vi "PDE_State_Machine_12_12_ver_3.vi"() -> ()   [LabVIEW 2017]
uses:
  SubVIs/FireSlider.ctl
  StateIndicator.ctl
  PDEState.ctl
  <vilib>/DAQmx/write.llb/DAQmx Write (Digital 1D Wfm NChan NSamp).vi
  <vilib>/DAQmx/read.llb/DAQmx Read (Analog 1D Wfm NChan NSamp).vi
  <vilib>/DAQmx/write.llb/DAQmx Write (Digital Wfm 1Chan NSamp).vi
  <vilib>/DAQmx/write.llb/DAQmx Write (Digital Bool 1Line 1Point).vi
  <vilib>/DAQmx/create/channels.llb/DAQmx Create Channel (AI-Current-Basic).vi
  <vilib>/DAQmx/create/channels.llb/DAQmx Create Channel (AI-Voltage-Basic).vi
  <vilib>/DAQmx/configure/timing.llb/DAQmx Timing (Sample Clock).vi
  <vilib>/DAQmx/create/channels.llb/DAQmx Create Channel (DO-Digital Output).vi
  <vilib>/DAQmx/create/channels.llb/DAQmx Create Channel (AI-Temperature-Thermocouple).vi
  <vilib>/Waveform/DWDTOps.llb/DWDT Uncompress Digital.vi
  <vilib>/DAQmx/miscellaneous.llb/DAQmx Fill In Error Info.vi
  <vilib>/Waveform/DTblOps.llb/DTbl Boolean Array to Digital.vi
  <resource>/objmgr/daqmx.rc
panel:
  out "PDE Sensors 2":T1 {"Downstream Oxygen" scale=0.0..150.0; "Upstream Oxygen" scale=0.0..150.0; "Fuel Pressure" scale=0.0..150.0}
  out "Predet Sensors 2":T2 {"Fuel Pressure" scale=0.0..150.0; "Oxidizer Pressure" scale=0.0..150.0}
  in  "Set_Oxygen_Pressure":bool
  in  "Save Data":bool
  in  "Filename":path=path "test.tdms"
  out "PDE Sensors":T1 {"Downstream Oxygen" scale=0.0..150.0; "Upstream Oxygen" scale=0.0..150.0; "Fuel Pressure" scale=0.0..150.0}
  in  "Predet Freq (Hz)":dbl=20.0 format="%#_13g"
  out "Predet Sensors":T2 {"Fuel Pressure" scale=0.0..150.0; "Oxidizer Pressure" scale=0.0..150.0}
  out "PDE Progress":dbl(slide) scale=0.0..1.0
  out "Predet Progress":dbl(slide) scale=0.0..1.0
  in  "Number of Predet Fires":T3=1 min=0 max=100 step=1 scale=1.0..100.0
  out "Predet Fire Counter":i32
  out "PDE State":T4 items=["Stop VI", "Predet Fire", "Control Button", "Stop", "Connecting", "Firing", "Testing ", "Idle", "Init"]
  in  "Number of Fires":T3=1 min=0 max=100 step=1 scale=1.0..100.0
  out "Fire Counter":i32
  in  "Predet Fire Button":bool
  in  "PDE Fire Button":bool
  in  "Test Button":bool
  in  "Go To Idle":bool
  in  "Abort VI":bool
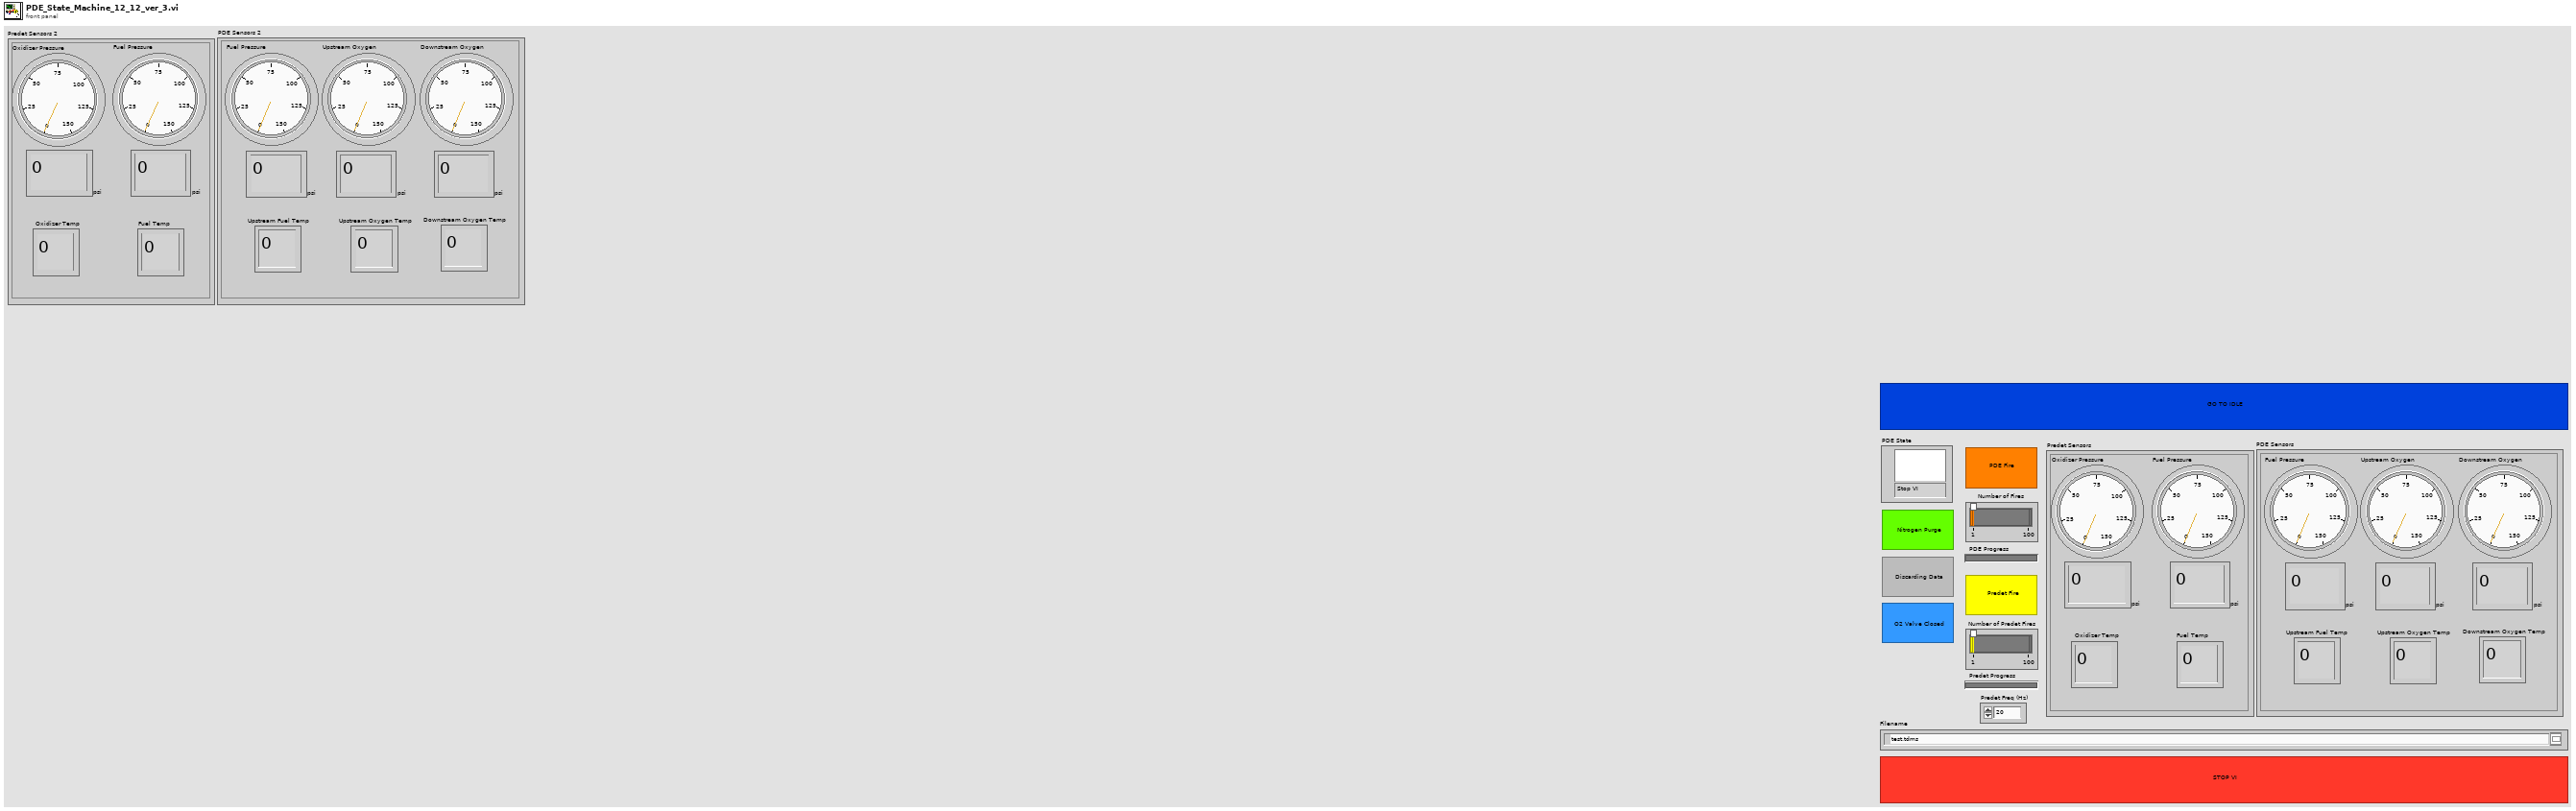
[diagram p1: front panel]
types:
  T1 = cluster{"Fuel Pressure":dbl, "Upstream Oxygen ":dbl, "Downstream Oxygen ":dbl, "Oxidizer Temp":dbl, "Oxidizer Temp 2":dbl, "Oxidizer Temp 3":dbl}
  T2 = cluster{"Oxidizer Pressure":dbl, "Fuel Pressure":dbl, "Oxidizer Temp":dbl, "Fuel Temp":dbl}
  T3 = typedef "FireSlider.ctl" = i32
  T4 = typedef "StateIndicator.ctl" = u16
  T5 = typedef "PDEState.ctl" = enum16{"Stop VI", "Predet Fire", "Control Button", "Stop", "Connecting", "Firing ", "Testing ", "Idle", "Init"}
  T6 = cluster{"Scalar":dbl, "Scalar":dbl, "Scalar":dbl, "Scalar":dbl, "Scalar":dbl, "Scalar":dbl}
  T7 = cluster{"Scalar":dbl, "Scalar":dbl, "Scalar":dbl, "Scalar":dbl}
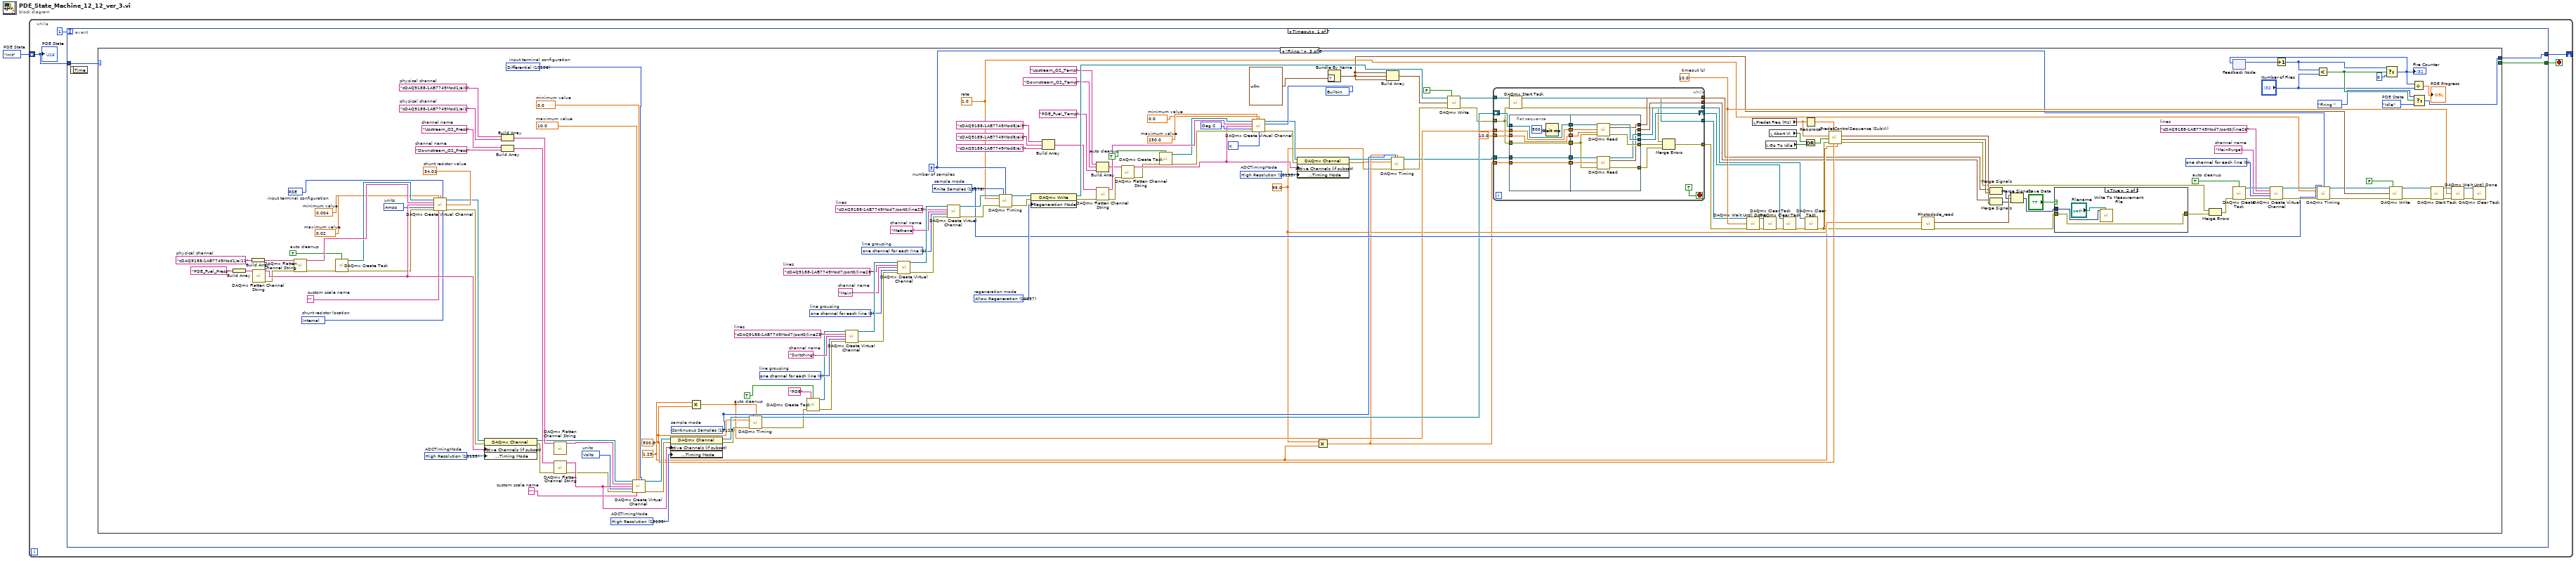
[diagram p0: block diagram]
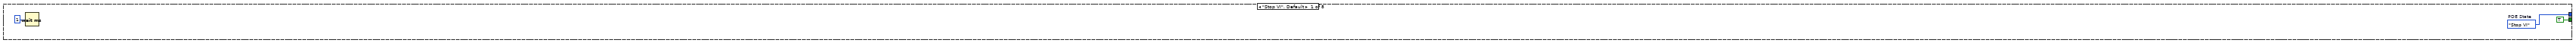
[diagram p2: hidden frame]
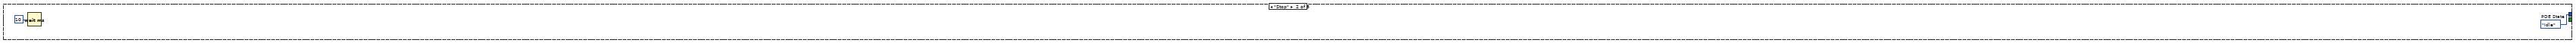
[diagram p3: hidden frame]
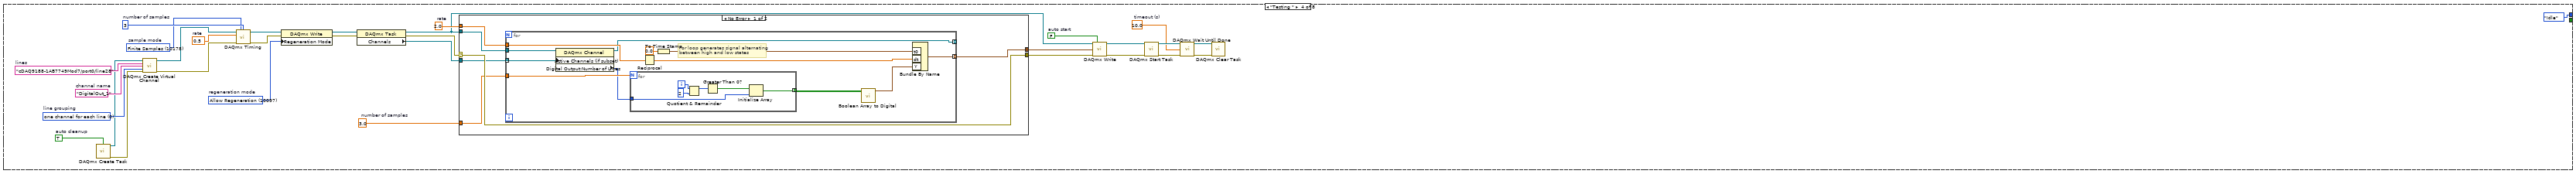
[diagram p5: hidden frame]
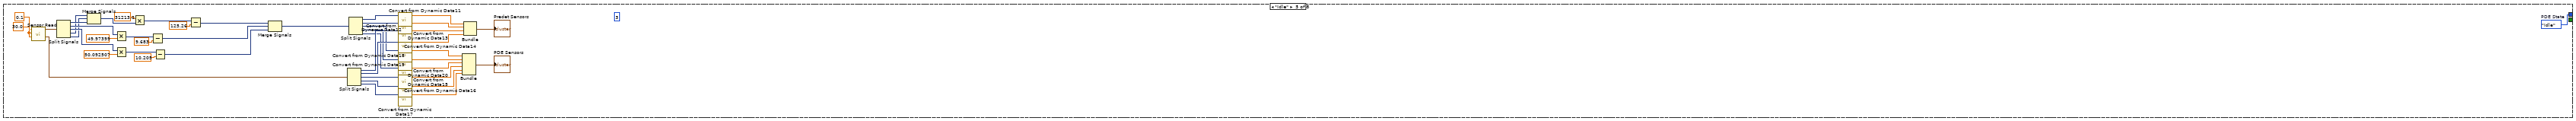
[diagram p7: hidden frame]
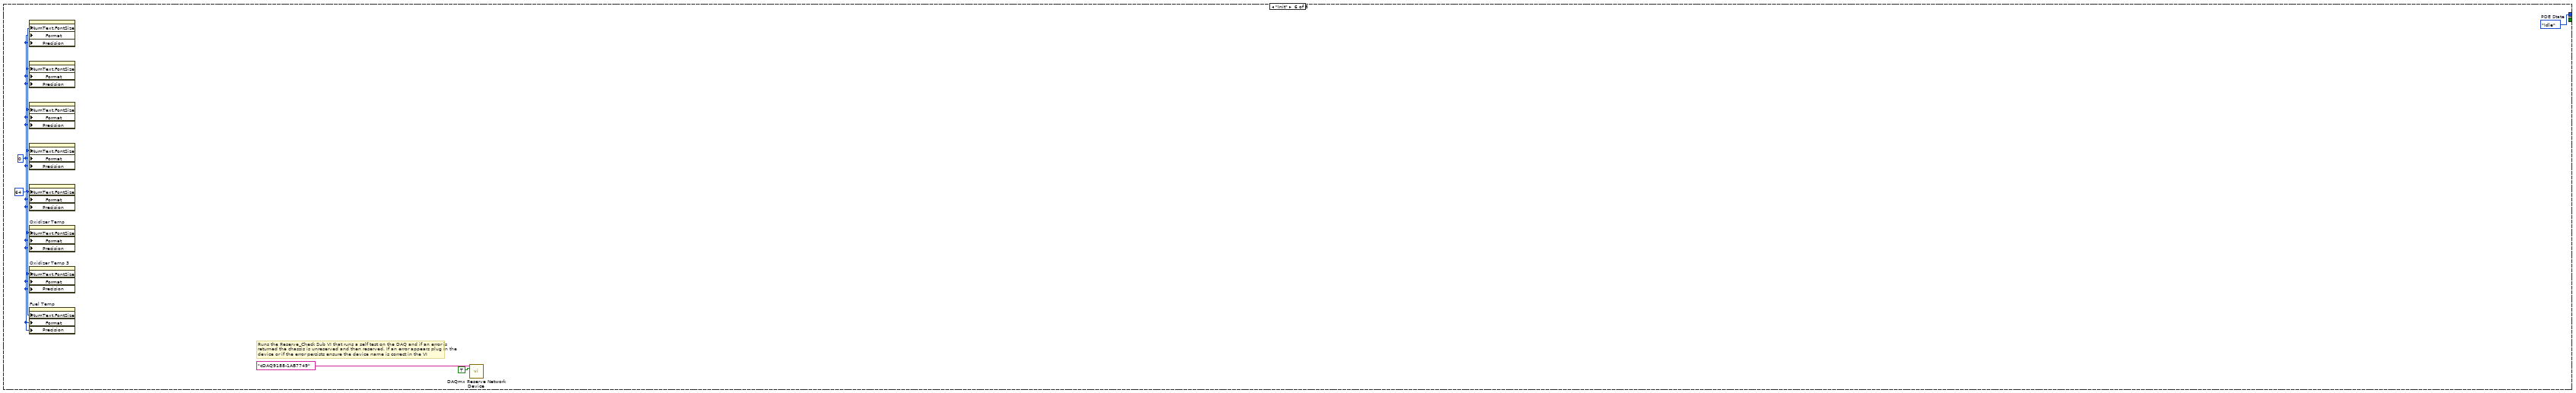
[diagram p8: hidden frame]
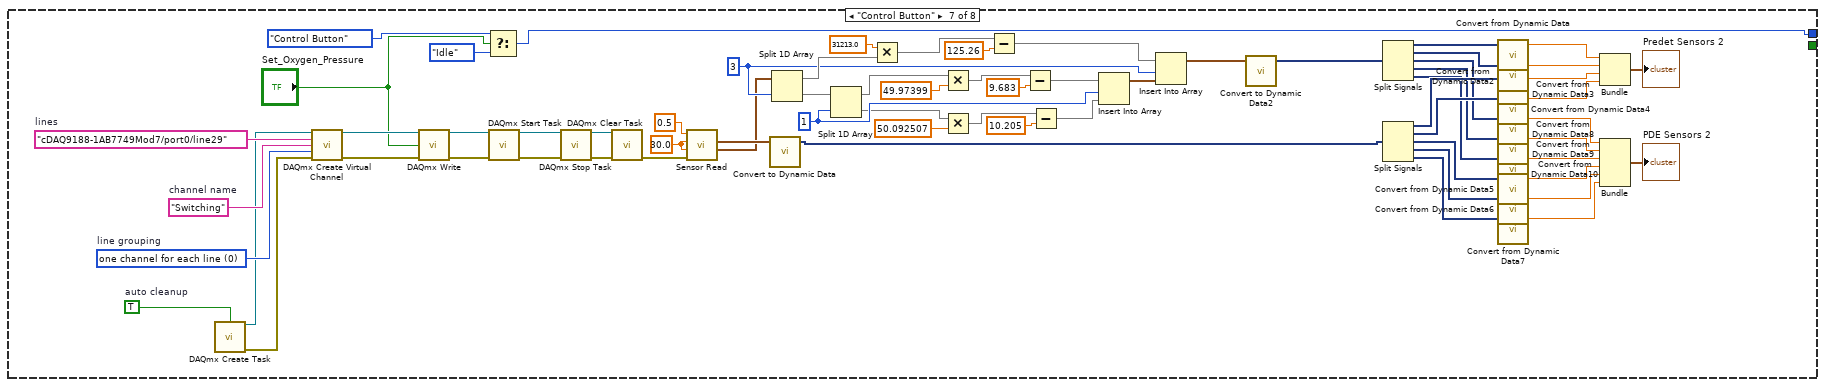
[diagram p9: hidden frame]
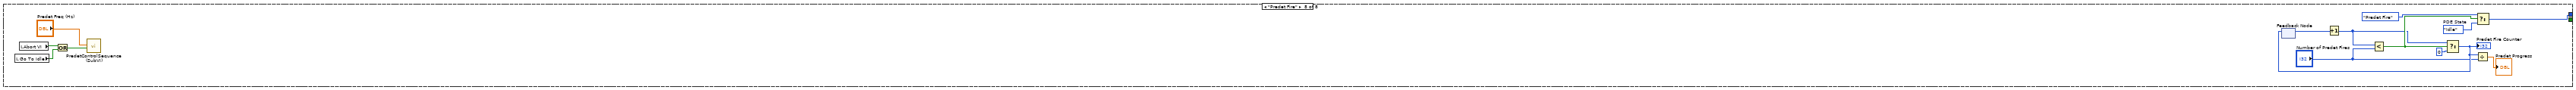
[diagram p10: hidden frame]
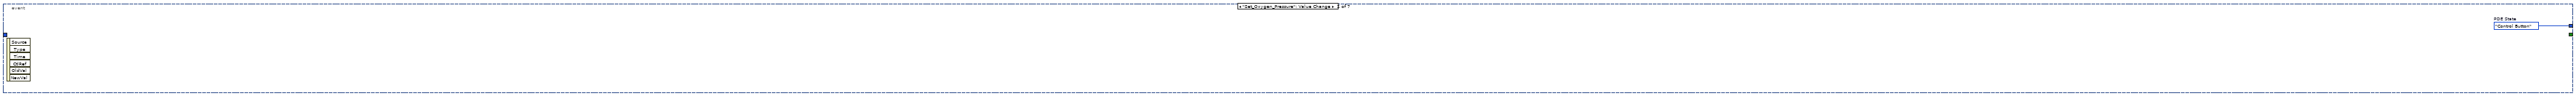
[diagram p11: hidden frame]
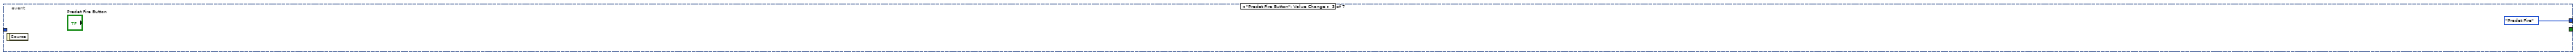
[diagram p12: hidden frame]
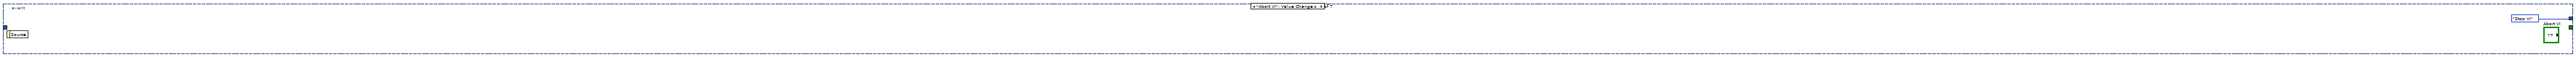
[diagram p13: hidden frame]
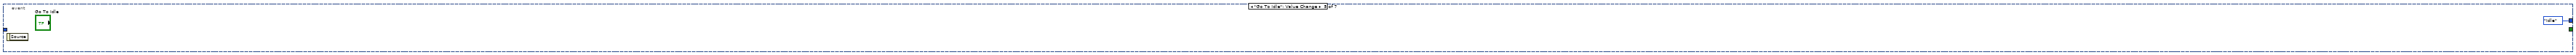
[diagram p14: hidden frame]
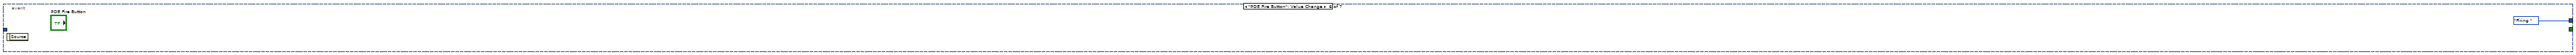
[diagram p15: hidden frame]
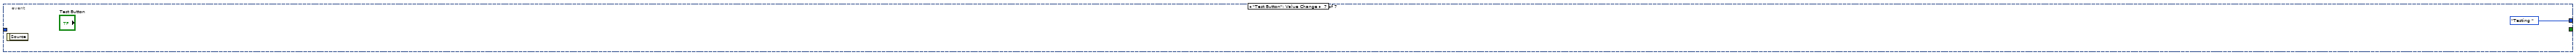
[diagram p16: hidden frame]
diagram:
  w1 = PDEState."Init"  # PDE State
  n1 = while {
    shift-right: [w4] -> _
    shift-left: w1 -> [w2]
    stop <- w3 stop-if-true
    n2 = event shown="[0] Timeout" {
      selector: _ -> [_ _ _ _ _ _ _]
      dyn-events: _ -> [_ _ _ _ _ _ _]
      timeout: 1 -> [_ _ _ _ _ _ _]
      tunnel: w2 -> [w8 _ _ _ _ _ _]
      tunnel: [w7 w415 PDEState."Predet Fire" ("PDE State") PDEState."Stop VI" ("PDE State") PDEState."Idle" ("PDE State") PDEState."Firing " ("PDE State") PDEState."Testing " ("PDE State")] -> w4
      tunnel: [w6 _ _ _ _ _ _] -> w3
      event Timeout {
        n3 = event-data() -> ()  [unwired: 1 in, 1 out]
        n4 = case shown="\"Firing \"" w8 {
          tunnel: [w11 w13 w175 PDEState."Idle" ("PDE State") w328 w333 w399 w408] -> w7
          tunnel: [TRUE _ _ _ _ _ _ _] -> w6
          frame "Stop VI", Default {
            w11 = PDEState."Stop VI"  # PDE State
            n5 = Wait (ms)(milliseconds to wait=u32 1 ("millisecond timer value")) -> ()  [unwired: 1 out]
          }
          frame "Stop" {
            w13 = PDEState."Idle"  # PDE State
            n6 = Wait (ms)(milliseconds to wait=u32 10 ("millisecond timer value")) -> ()  [unwired: 1 out]
          }
          frame "Firing " {
            w89 = 10195 items=["High Resolution"=10195, "High Speed"=14712, "Best 50 Hz Rejection"=14713, "Best 60 Hz Rejection"=14714]  # ADCTimingMode
            w100 = "Downstream_O2_Press"  # channel name
            w97 = "cDAQ9188-1AB7749Mod1/ai1"  # physical channel
            w88 = 10106 items=["default"=-1, "RSE"=10083, "NRSE"=10078, "Differential"=10106, "Pseudodifferential"=12529]  # input terminal configuration
            w102 = 10348 items=["Volts"=10348, "From Custom Scale"=10065]  # units
            w101 = "Upstream_O2_Press"  # channel name
            w87 = ""  # custom scale name
            w86 = 0.0  # minimum value
            w85 = 10.0  # maximum value
            w96 = "cDAQ9188-1AB7749Mod1/ai0"  # physical channel
            w83 = "cDAQ9188-1AB7749Mod1/ai11"  # physical channel
            w90 = 10123 items=["Finite Samples"=10178, "Continuous Samples"=10123, "Hardware Timed Single Point"=12522]  # sample mode
            w63 = 10195 items=["High Resolution"=10195, "High Speed"=14712, "Best 50 Hz Rejection"=14713, "Best 60 Hz Rejection"=14714]  # ADCTimingMode
            w64 = 10083 items=["default"=-1, "RSE"=10083, "NRSE"=10078, "Differential"=10106, "Pseudodifferential"=12529]  # input terminal configuration
            w65 = 10342 items=["Amps"=10342, "From Custom Scale"=10065]  # units
            w66 = 34.01  # shunt resistor value
            w67 = 10200 items=["Internal"=10200, "External"=10167]  # shunt resistor location
            w69 = ""  # custom scale name
            w70 = 0.004  # minimum value
            w71 = 0.02  # maximum value
            w73 = TRUE  # auto cleanup
            w60 = 10143 items=["Deg C"=10143, "Deg F"=10144, "Kelvins"=10325, "Deg R"=10145, "From Custom Scale"=10065] ("units")
            w59 = 10073 items=["J"=10072, "K"=10073, "N"=10077, "R"=10082, "S"=10085, "T"=10086, "B"=10047, "E"=10055] ("thermocouple type")
            w58 = 10200 items=["Built-In"=10200, "Constant Value"=10116, "Channel"=10113] ("cjc source")
            w49 = 10195 items=["High Resolution"=10195, "High Speed"=14712, "Best 50 Hz Rejection"=14713, "Best 60 Hz Rejection"=14714]  # ADCTimingMode
            w52 = 0.0  # minimum value
            w53 = 250.0  # maximum value
            w55 = TRUE  # auto cleanup
            w34 = 1.25 ("Sampling Time")
            w35 = 95.0 ("Temperature Freq")
            w36 = 500.0 ("Pressure Freq")
            w130 = 0 items=["one channel for each line", "one channel for all lines"] ("line grouping")
            w136 = 0 items=["one channel for each line", "one channel for all lines"]  # line grouping
            w135 = "Methane"  # channel name
            w137 = "cDAQ9188-1AB7749Mod7/port0/line25"  # lines
            w141 = 0 items=["one channel for each line", "one channel for all lines"]  # line grouping
            w140 = "Main"  # channel name
            w142 = "cDAQ9188-1AB7749Mod7/port0/line28"  # lines
            w146 = 0 items=["one channel for each line", "one channel for all lines"]  # line grouping
            w145 = "Switching"  # channel name
            w147 = "cDAQ9188-1AB7749Mod7/port0/line29"  # lines
            w161 = TRUE  # auto cleanup
            w156 = "MainPurge"  # channel name
            w157 = "cDAQ9188-1AB7749Mod7/port0/line26"  # lines
            w168 = 10097 items=["Allow Regeneration"=10097, "Do Not Allow Regeneration"=10158]  # regeneration mode
            w123 = 10178 items=["Finite Samples"=10178, "Continuous Samples"=10123, "Hardware Timed Single Point"=12522]  # sample mode
            w124 = 3  # number of samples
            w122 = 1.0  # rate
            w170 = TRUE  # auto cleanup
            w148 = 10.0  # timeout (s)
            w176 = PDEState."Idle"  # PDE State
            n7 = Build Array("PDE_Fuel_Press" ("element")) -> (w76:string[])
            n8 = Build Array(w83) -> (w78:string[])
            n9 = call <vilib>:"DAQmx Flatten Channel String.vi"("names in"=w76) -> ("names out"=w77:string, "error out"=w38:errorcluster)  [unwired: 13 in]
            n10 = call <vilib>:"DAQmx Flatten Channel String.vi"("names in"=w78, "error in"=w38) -> ("names out"=w75:string, "error out"=w16:errorcluster)  [unwired: 12 in]
            n11 = call <vilib>:"DAQmx Create Task.vi"("auto cleanup"=w73, "error in"=w16) -> ("task out"=w72:refnum<k21>, "error out"=w74:errorcluster)  [unwired: 3 in, 9 out]
            n12 = call-poly <vilib>:"DAQmx Create Virtual Channel.vi"("task in"=w72, "maximum value"=w71, "minimum value"=w70, "input terminal configuration"=w64, "physical channels"=w75, "name to assign"=w77, "external shunt resistor value"=w66, "units"=w65, "error in"=w74, "custom scale name"=w69, "shunt resistor location"=w67) -> ("task out"=w62:refnum<k21>, "error out"=w68:errorcluster)  [unwired: 3 out]
            n13 = property class="DAQmx Channel"(reference=w62, error in=w68, "Active Channels (if subset)"=w77, "Analog Input:General Properties:Digitizer/ADC:Timing Mode"=w63) -> (reference out=w92:refnum<k21>, error out=w18:errorcluster)
            n14 = Build Array(w96, w97) -> (w95:string[])
            n15 = Build Array(w101, w100) -> (w99:string[])
            n16 = call <vilib>:"DAQmx Flatten Channel String.vi"("names in"=w95) -> ("names out"=w98:string)  [unwired: 13 in, 1 out]
            n17 = call <vilib>:"DAQmx Flatten Channel String.vi"("names in"=w99, "error in"=w18) -> ("names out"=w105:string, "error out"=w17:errorcluster)  [unwired: 12 in]
            n18 = call-poly <vilib>:"DAQmx Create Virtual Channel.vi"("task in"=w92, "maximum value"=w85, "minimum value"=w86, "input terminal configuration"=w88, "physical channels"=w98, "name to assign"=w105, "units"=w102, "error in"=w17, "custom scale name"=w87) -> ("task out"=w103:refnum<k21>, "error out"=w104:errorcluster)  [unwired: 5 in]
            n19 = property class="DAQmx Channel"(reference=w103, error in=w104, "Active Channels (if subset)"=w105, "Analog Input:General Properties:Digitizer/ADC:Timing Mode"=w89) -> (reference out=w91:refnum<k21>, error out=w93:errorcluster)
            n20 = Multiply(x=w34, y=w36) -> (x*y=w39:dbl)
            n21 = call-poly <vilib>:"DAQmx Timing.vi"("task/channels in"=w91, "sample mode"=w90, "samples per channel"=w39, "rate"=w36, "error in"=w93) -> ("task out"=w79:refnum<k21>, "error out"=w22:errorcluster)  [unwired: 2 in, 7 out]
            n22 = call <vilib>:"DAQmx Create Task.vi"("new task name"="PDE", "auto cleanup"=w170, "error in"=w22) -> ("task out"=w131:refnum<k21>, "error out"=w132:errorcluster)  [unwired: 11 in]
            n23 = call-poly <vilib>:"DAQmx Create Virtual Channel.vi"("task in"=w131, "lines"=w147, "name to assign"=w145, "line grouping"=w146, "error in"=w132) -> ("task out"=w143:refnum<k21>, "error out"=w144:errorcluster)  [unwired: 9 in]
            n24 = call-poly <vilib>:"DAQmx Create Virtual Channel.vi"("task in"=w143, "lines"=w142, "name to assign"=w140, "line grouping"=w141, "error in"=w144) -> ("task out"=w138:refnum<k21>, "error out"=w139:errorcluster)  [unwired: 9 in]
            n25 = call-poly <vilib>:"DAQmx Create Virtual Channel.vi"("task in"=w138, "lines"=w137, "name to assign"=w135, "line grouping"=w136, "error in"=w139) -> ("task out"=w133:refnum<k21>, "error out"=w134:errorcluster)  [unwired: 9 in]
            n26 = call-poly <vilib>:"DAQmx Timing.vi"("task/channels in"=w133, "sample mode"=w123, "samples per channel"=w124, "rate"=w122, "error in"=w134) -> ("task out"=w169:refnum<k21>, "error out"=w21:errorcluster)  [unwired: 9 in]
            n27 = property class="DAQmx Write"(reference=w169, error in=w21, "Regeneration Mode"=w168) -> (reference out=w167:refnum<k21>, error out=w20:errorcluster)
            n28 = Build Array("cDAQ9188-1AB7749Mod8/ai5" ("element"), "cDAQ9188-1AB7749Mod8/ai6" ("element"), "cDAQ9188-1AB7749Mod8/ai7" ("element")) -> (w61:string[])
            n29 = Build Array("Upstream_O2_Temp" ("name to assign"), "Downstream_O2_Temp" ("name to assign"), "PDE_Fuel_Temp" ("name to assign")) -> (w45:string[])
            n30 = call <vilib>:"DAQmx Flatten Channel String.vi"("names in"=w61, "error in"=w20) -> ("names out"=w57:string, "error out"=w37:errorcluster)  [unwired: 12 in]
            n31 = call <vilib>:"DAQmx Flatten Channel String.vi"("names in"=w45, "error in"=w37) -> ("names out"=w41:string, "error out"=w40:errorcluster)  [unwired: 12 in]
            n32 = call <vilib>:"DAQmx Create Task.vi"("auto cleanup"=w55, "error in"=w40) -> ("task out"=w54:refnum<k21>, "error out"=w56:errorcluster)  [unwired: 3 in, 9 out]
            n33 = call-poly <vilib>:"DAQmx Create Virtual Channel.vi"("task in"=w54, "maximum value"=w53, "minimum value"=w52, "physical channels"=w57, "cjc source"=w58, "name to assign"=w41, "units"=w60, "error in"=w56, "thermocouple type"=w59) -> ("task out"=w48:refnum<k21>, "error out"=w51:errorcluster)  [unwired: 5 in]
            n34 = property class="DAQmx Channel"(reference=w48, error in=w51, "Active Channels (if subset)"=w41, "Analog Input:General Properties:Digitizer/ADC:Timing Mode"=w49) -> (reference out=w47:refnum<k21>, error out=w50:errorcluster)
            n35 = Multiply(x=w35, y=w34) -> (x*y=w31:dbl)
            n36 = Bundle By Name("Y"=digitaldata {"transitions"=[], "data"=[[0], [1], [0]]}) -> (w129:digitalwaveform)  [unwired: 1 in]
            n37 = Build Array(w129, w129, w129) -> (w165:digitalwaveform[])
            n38 = call-poly <vilib>:"DAQmx Timing.vi"("task/channels in"=w47, "sample mode"=w90, "samples per channel"=w31, "rate"=w35, "error in"=w50) -> ("task out"=w33:refnum<k21>, "error out"=w19:errorcluster)  [unwired: 2 in, 7 out]
            n39 = call-poly <vilib>:"DAQmx Write.vi"("task/channels in"=w167, "auto start"=FALSE, "data"=w165, "error in"=w19) -> ("task out"=w25:refnum<k21>, "error out"=w28:errorcluster)  [unwired: 9 in, 1 out]
            n40 = while {
              tunnel: 10.0 ("timeout") -> [w202]
              tunnel: w39 -> [w199]
              shift-right: [w201] -> w46
              shift-left: w79 -> [w200]
              tunnel: w33 -> [w198]
              tunnel: [w195] -> w32
              tunnel: w31 -> [w194]
              tunnel: [w193] -> w30
              tunnel: [w192] -> w29
              tunnel: [w189] -> w26
              tunnel: w25 -> [w188]
              tunnel: [w187] -> w15
              tunnel: w28 -> [w186]
              stop <- TRUE stop-if-true
              n41 = call <vilib>:"DAQmx Start Task.vi"("task/channels in"=w188, "error in"=w186) -> ("task out"=w189:refnum<k21>, "error out"=w190:errorcluster)  [unwired: 12 in]
              n42 = flat-sequence {
                tunnel: w186 -> [w205]
                tunnel: w194 -> [w204]
                tunnel: w198 -> [w206]
                tunnel: w199 -> [w207]
                tunnel: w200 -> [w208]
                tunnel: w202 -> [w209]
                tunnel: [w209] -> w185
                tunnel: [w208] -> w184
                tunnel: [w207] -> w183
                tunnel: [w206] -> w182
                tunnel: [w204] -> w181
                tunnel: [w205] -> w180
                tunnel: [w220] -> w201
                tunnel: [w216] -> w197
                tunnel: [w215] -> w196
                tunnel: [w214] -> w195
                tunnel: [w212] -> w193
                tunnel: [w211] -> w192
                tunnel: w185 -> [w221]
                tunnel: w184 -> [w219]
                tunnel: w183 -> [w218]
                tunnel: w182 -> [w217]
                tunnel: w181 -> [w213]
                tunnel: w180 -> [w210]
                frame #0 {
                  n43 = Wait (ms)(milliseconds to wait=u32 500) -> ()  [unwired: 1 out]
                }
                frame #1 {
                  n44 = call-poly <vilib>:"DAQmx Read.vi"("task/channels in"=w219, "number of samples per channel"=w218, "timeout"=w221, "error in"=w210) -> ("task out"=w220:refnum<k21>, "data"=w211:waveform(dbl)[], "error out"=w216:errorcluster)  [unwired: 9 out]
                  n45 = call-poly <vilib>:"DAQmx Read.vi"("task/channels in"=w217, "number of samples per channel"=w213, "error in"=w210) -> ("task out"=w214:refnum<k21>, "data"=w212:waveform(dbl)[], "error out"=w215:errorcluster)  [unwired: 1 in, 9 out]
                }
              }
              n46 = Merge Errors(w190, w197, w196) -> (w187:errorcluster)
            }
            n47 = call <vilib>:"DAQmx Wait Until Done.vi"("task/channels in"=w26, "timeout (sec)"=w148, "error in"=w15) -> ("task out"=w160:refnum<k21>, "error out"=w171:errorcluster)  [unwired: 11 in]
            n48 = local read "Predet Freq (Hz)"() -> (w116:dbl)
            n49 = call <vilib>:"DAQmx Clear Task.vi"("task in"=w160, "error in"=w171) -> ("error out"=w24:errorcluster)  [unwired: 13 in]
            n50 = local read "Go To Idle"() -> (w163:bool)
            n51 = local read "Abort VI"() -> (w164:bool)
            n52 = call <vilib>:"DAQmx Clear Task.vi"("task in"=w46, "error in"=w24) -> ("error out"=w23:errorcluster)  [unwired: 13 out]
            n53 = Or(x=w164, y=w163) -> (x .or. y?=w162:bool)
            n54 = Reciprocal(x=w116) -> (1/x=w106:dbl)
            n55 = call <vilib>:"DAQmx Clear Task.vi"("task in"=w32, "error in"=w23) -> ("error out"=w14:errorcluster)  [unwired: 13 out]
            n56 = call "PredetControlSequence (SubVI).vi"("Temperature Freq"=w35, "Pressure Freq"=w36, "Sampling Time"=w106, "Error In"=w14, "Stop Button"=w162, "Predet Freq (Hz)"=w116) -> ("Error Out"=w107:errorcluster, "Pressure Data"=w109:waveform(dbl)[], "Temperature Data"=w108:waveform(dbl)[])  [unwired: 2 in, 1 out]
            n57 = call "Photodode_read.vi"("Error In"=w14, "Sampling Time"=w34) -> ("error out"=w110:errorcluster, "data"=w115:waveform(dbl)[])  [unwired: 6 in]
            n58 = Merge Signals(w29, w109) -> (w114:dynamicdata)
            n59 = Merge Signals(w30, w108) -> (w113:dynamicdata)
            n60 = Merge Signals(w115, w114, w113) -> (w111:dynamicdata)
            n61 = case shown="True" "Save Data" {
              tunnel: w111 -> [_ w225]
              tunnel: w110 -> [w222 w223]
              tunnel: [w222 w223] -> w117
              frame False {
              }
              frame True {
                n62 = call "Write To Measurement File"("Signals"=w225, "Filename"="Filename") -> ()  [unwired: 15 in, 3 out]
              }
            }
            n63 = Merge Errors(w107, w117) -> (w119:errorcluster)
            n64 = feedback #1() -> (w120:i32)  [unwired: 1 in]
            n65 = call <vilib>:"DAQmx Create Task.vi"("auto cleanup"=w161, "error in"=w119) -> ("task out"=w159:refnum<k21>, "error out"=w158:errorcluster)  [unwired: 12 in]
            n66 = call-poly <vilib>:"DAQmx Create Virtual Channel.vi"("task in"=w159, "lines"=w157, "name to assign"=w156, "line grouping"=w130, "error in"=w158) -> ("task out"=w128:refnum<k21>, "error out"=w125:errorcluster)  [unwired: 9 in]
            n67 = Increment(x=w120) -> (x+1=w121:i32)
            n68 = Less?(x=w121, y="Number of Fires") -> (x < y?=w179:bool)
            n69 = call-poly <vilib>:"DAQmx Timing.vi"("task/channels in"=w128, "sample mode"=w123, "samples per channel"=w124, "rate"=w122, "error in"=w125) -> ("task out"=w127:refnum<k21>, "error out"=w126:errorcluster)  [unwired: 9 in]
            n70 = Select(t=w121, s=w179, f=0 ("s? t:f")) -> (s? t:f=w173:i32)
            "Fire Counter" <- w173
            n71 = feedback-in #1(w173) -> ()
            n72 = call-poly <vilib>:"DAQmx Write.vi"("task/channels in"=w127, "auto start"=FALSE, "data"=w129, "error in"=w126) -> ("task out"=w149:refnum<k21>, "error out"=w150:errorcluster)  [unwired: 9 in, 1 out]
            n73 = Divide(x=w173, y="Number of Fires") -> (x/y=→"PDE Progress":dbl)
            n74 = Select(t=PDEState."Firing ", s=w179, f=w176) -> (s? t:f=w175:T5)
            n75 = call <vilib>:"DAQmx Start Task.vi"("task/channels in"=w149, "error in"=w150) -> ("task out"=w152:refnum<k21>, "error out"=w154:errorcluster)  [unwired: 12 in]
            n76 = call <vilib>:"DAQmx Wait Until Done.vi"("task/channels in"=w152, "timeout (sec)"=w148, "error in"=w154) -> ("task out"=w151:refnum<k21>, "error out"=w153:errorcluster)  [unwired: 11 in]
            n77 = call <vilib>:"DAQmx Clear Task.vi"("task in"=w151, "error in"=w153) -> ()  [unwired: 13 in, 1 out]
          }
          frame "Testing " {
            w237 = 10097 items=["Allow Regeneration"=10097, "Do Not Allow Regeneration"=10158]  # regeneration mode
            w239 = 10178 items=["Finite Samples"=10178, "Continuous Samples"=10123, "Hardware Timed Single Point"=12522]  # sample mode
            w240 = 3  # number of samples
            w241 = 0.5  # rate
            w246 = 0 items=["one channel for each line", "one channel for all lines"]  # line grouping
            w245 = "DigitalOut_1"  # channel name
            w247 = "cDAQ9188-1AB7749Mod7/port0/line28"  # lines
            w248 = TRUE  # auto cleanup
            w249 = 10.0  # timeout (s)
            w233 = 2.0  # rate
            w234 = 3.0  # number of samples
            w256 = FALSE  # auto start
            n78 = call <vilib>:"DAQmx Create Task.vi"("auto cleanup"=w248) -> ("task out"=w227:refnum<k21>, "error out"=w226:errorcluster)  [unwired: 13 in]
            n79 = call-poly <vilib>:"DAQmx Create Virtual Channel.vi"("task in"=w227, "lines"=w247, "name to assign"=w245, "line grouping"=w246, "error in"=w226) -> ("task out"=w242:refnum<k21>, "error out"=w244:errorcluster)  [unwired: 9 in]
            n80 = call-poly <vilib>:"DAQmx Timing.vi"("task/channels in"=w242, "sample mode"=w239, "samples per channel"=w240, "rate"=w241, "error in"=w244) -> ("task out"=w238:refnum<k21>, "error out"=w243:errorcluster)  [unwired: 9 in]
            n81 = property class="DAQmx Write"(reference=w238, error in=w243, "Regeneration Mode"=w237) -> (reference out=w230:refnum<k21>, error out=w229:errorcluster)
            n82 = property class="DAQmx Task"(reference=w230, error in=w229) -> (reference out=w228:refnum<k21>, error out=w235:errorcluster, "Channels"=w236:refnum<k21>[])
            n83 = case shown="No Error" w235 {
              selector: w235 -> [w261 w282]
              tunnel: w233 -> [w263 _]
              tunnel: [w262 _] -> w232
              tunnel: [w261 w282] -> w231
              tunnel: w234 -> [w260 _]
              tunnel: w236 -> [w259 _]
              tunnel: w228 -> [w258 _]
              frame No Error {
                n84 = for {
                  tunnel: w263 -> [w275]
                  tunnel: [w270] -> w262 mode=indexing
                  tunnel: w260 -> [w269]
                  tunnel: w259 -> [w267] mode=indexing
                  tunnel: w258 -> [w265]
                  tunnel: [w264] -> _ mode=indexing
                  # "For loop generates signal alternating\nbetween high and low states"
                  n85 = property class="DAQmx Channel"(reference=w265, "Active Channels (if subset)"=w267) -> (reference out=w264:refnum<k21>, "Digital Output:Number of Lines"=w266:u32)  [unwired: 1 in, 1 out]
                  n86 = for {
                    N: w269 -> [_]
                    tunnel: [w276] -> w268 mode=indexing
                    tunnel: w266 -> [w277]
                    i -> [w281]
                    n87 = Quotient & Remainder(x=w281, y=2) -> (x-y*floor(x/y)=w279:i32)  [unwired: 1 out]
                    n88 = Greater Than 0?(x=w279) -> (x > 0?=w278:bool)
                    n89 = Initialize Array(w278, w277) -> (w276:bool[])
                  }
                  n90 = Reciprocal(x=w275) -> (1/x=w271:dbl)
                  n91 = To Time Stamp(1:0.0) -> (0:w273:timestamp)
                  n92 = call-poly <vilib>:"Boolean Array to Digital.vi"("boolean array"=w268) -> ("digital data"=w272:digitaldata)  [unwired: 3 in, 7 out]
                  n93 = Bundle By Name("t0"=w273, "dt"=w271, "Y"=w272) -> (w270:digitalwaveform)  [unwired: 1 out]
                }
              }
              frame Error {
              }
            }
            n94 = call-poly <vilib>:"DAQmx Write.vi"("task/channels in"=w228, "auto start"=w256, "data"=w232, "error in"=w231) -> ("task out"=w252:refnum<k21>, "error out"=w251:errorcluster)  [unwired: 9 in, 1 out]
            n95 = call <vilib>:"DAQmx Start Task.vi"("task/channels in"=w252, "error in"=w251) -> ("task out"=w255:refnum<k21>, "error out"=w254:errorcluster)  [unwired: 12 in]
            n96 = call <vilib>:"DAQmx Wait Until Done.vi"("task/channels in"=w255, "timeout (sec)"=w249, "error in"=w254) -> ("task out"=w250:refnum<k21>, "error out"=w253:errorcluster)  [unwired: 11 in]
            n97 = call <vilib>:"DAQmx Clear Task.vi"("task in"=w250, "error in"=w253) -> ()  [unwired: 13 in, 1 out]
          }
          frame "Idle" {
            (unwired) 3 ("index")
            w306 = 30.0 ("Pressure Freq")
            w328 = PDEState."Idle"  # PDE State
            n98 = call "Sensor Read.vi"("Pressure Freq"=w306, "Temperature Freq"=w306, "Sampling Time"=0.1) -> ("Temperature Data"=w304:waveform(dbl)[], "Pressure Data"=w302:waveform(dbl)[])  [unwired: 5 in, 2 out]
            n99 = Split Signals(w302) -> (w286:dynamicdata, w291:dynamicdata, w290:dynamicdata, w285:dynamicdata, w284:dynamicdata)  [unwired: 5 in]
            n100 = Merge Signals(w285, w284, w286) -> (w298:dynamicdata)
            n101 = Multiply(x=w291, y=49.97399) -> (x*y=w294:dynamicdata)
            n102 = Multiply(x=w290, y=50.092507) -> (x*y=w297:dynamicdata)
            n103 = Multiply(x=31213.0, y=w298) -> (x*y=w299:dynamicdata)
            n104 = Subtract(x=w294, y=9.683) -> (x-y=w288:dynamicdata)
            n105 = Subtract(x=w297, y=10.205) -> (x-y=w287:dynamicdata)
            n106 = Subtract(x=w299, y=125.26) -> (x-y=w289:dynamicdata)
            n107 = Merge Signals(w289, w288, w287) -> (w283:dynamicdata)
            n108 = Split Signals(w304) -> (w324:dynamicdata, w326:dynamicdata, w321:dynamicdata, w320:dynamicdata, w319:dynamicdata)  [unwired: 5 in]
            n109 = Split Signals(w283) -> (w313:dynamicdata, w312:dynamicdata, w311:dynamicdata, w310:dynamicdata, w309:dynamicdata)  [unwired: 5 in]
            n110 = call "Convert from Dynamic Data11"("Dynamic Data Type"=w313) -> ("Scalar"=w323:dbl)  [unwired: 3 in]
            n111 = call "Convert from Dynamic Data12"("Dynamic Data Type"=w312) -> ("Scalar"=w322:dbl)  [unwired: 3 in]
            n112 = call "Convert from Dynamic Data13"("Dynamic Data Type"=w324) -> ("Scalar"=w325:dbl)  [unwired: 3 in]
            n113 = call "Convert from Dynamic Data14"("Dynamic Data Type"=w326) -> ("Scalar"=w327:dbl)  [unwired: 3 in]
            n114 = call "Convert from Dynamic Data18"("Dynamic Data Type"=w311) -> ("Scalar"=w316:dbl)  [unwired: 3 in]
            n115 = call "Convert from Dynamic Data19"("Dynamic Data Type"=w310) -> ("Scalar"=w317:dbl)  [unwired: 3 in]
            n116 = call "Convert from Dynamic Data20"("Dynamic Data Type"=w309) -> ("Scalar"=w318:dbl)  [unwired: 3 in]
            n117 = call "Convert from Dynamic Data15"("Dynamic Data Type"=w321) -> ("Scalar"=w315:dbl)  [unwired: 3 in]
            n118 = call "Convert from Dynamic Data16"("Dynamic Data Type"=w320) -> ("Scalar"=w314:dbl)  [unwired: 3 in]
            n119 = call "Convert from Dynamic Data17"("Dynamic Data Type"=w319) -> ("Scalar"=w303:dbl)  [unwired: 3 in]
            n120 = Bundle("Scalar"=w316, "Scalar"=w317, "Scalar"=w318, "Scalar"=w315, "Scalar"=w314, "Scalar"=w303) -> (→"PDE Sensors":T6)  [unwired: 1 in]
            n121 = Bundle("Scalar"=w323, "Scalar"=w322, "Scalar"=w325, "Scalar"=w327) -> (→"Predet Sensors":T7)  [unwired: 1 in]
          }
          frame "Init" {
            w329 = u8 0 ("Display Format:Format")
            w330 = u32 64 ("Numeric Text.Font:Size")
            w333 = PDEState."Idle"  # PDE State
            # "Runs the Reserve_Check Sub VI that runs a self test on the DAQ and if an error is returned the chassis is unreserved and then reserved. If an error appears plug in the device or if the error persists ensure the device name is correct in the VI"
            n122 = property class="DigNum (strict)"("NumText.FontSize"=w330, "Format"=w329, "Precision"=w329) -> ()  [unwired: 2 in, 2 out]
            n123 = property class="DigNum (strict)"("NumText.FontSize"=w330, "Format"=w329, "Precision"=w329) -> ()  [unwired: 2 in, 2 out]
            n124 = property class="DigNum (strict)"("NumText.FontSize"=w330, "Format"=w329, "Precision"=w329) -> ()  [unwired: 2 in, 2 out]
            n125 = property class="DigNum (strict)"("NumText.FontSize"=w330, "Format"=w329, "Precision"=w329) -> ()  [unwired: 2 in, 2 out]
            n126 = property class="DigNum (strict)"("NumText.FontSize"=w330, "Format"=w329, "Precision"=w329) -> ()  [unwired: 2 in, 2 out]
            n127 = property on="Oxidizer Temp" class="DigNum (strict)"("NumText.FontSize"=w330, "Format"=w329, "Precision"=w329) -> ()  [unwired: 2 in, 2 out]
            n128 = property on="Oxidizer Temp 3" class="DigNum (strict)"("NumText.FontSize"=w330, "Format"=w329, "Precision"=w329) -> ()  [unwired: 2 in, 2 out]
            n129 = property on="Fuel Temp" class="DigNum (strict)"("NumText.FontSize"=w330, "Format"=w329, "Precision"=w329) -> ()  [unwired: 2 in, 2 out]
            n130 = call <vilib>:"DAQmx Reserve Network Device.vi"("device in"=tag "cDAQ9188-1AB7749", "override reservation?"=TRUE) -> ()  [unwired: 12 in, 2 out]
          }
          frame "Control Button" {
            w349 = 0 items=["one channel for each line", "one channel for all lines"]  # line grouping
            w348 = "Switching"  # channel name
            w350 = "cDAQ9188-1AB7749Mod7/port0/line29"  # lines
            w351 = TRUE  # auto cleanup
            w335 = 30.0 ("Sampling Frequency")
            w362 = 1 ("index")
            w365 = 3 ("index")
            n131 = call <vilib>:"DAQmx Create Task.vi"("auto cleanup"=w351) -> ("task out"=w347:refnum<k21>, "error out"=w346:errorcluster)  [unwired: 13 in]
            n132 = call-poly <vilib>:"DAQmx Create Virtual Channel.vi"("task in"=w347, "lines"=w350, "name to assign"=w348, "line grouping"=w349, "error in"=w346) -> ("task out"=w345:refnum<k21>, "error out"=w344:errorcluster)  [unwired: 9 in]
            n133 = call-poly <vilib>:"DAQmx Write.vi"("task/channels in"=w345, "data"="Set_Oxygen_Pressure", "error in"=w344) -> ("task out"=w342:refnum<k21>, "error out"=w341:errorcluster)  [unwired: 10 in, 1 out]
            n134 = Select(t=PDEState."Control Button" ("PDE State"), s="Set_Oxygen_Pressure", f=PDEState."Idle" ("PDE State")) -> (s? t:f=w399:T5)
            n135 = call <vilib>:"DAQmx Start Task.vi"("task/channels in"=w342, "error in"=w341) -> ("task out"=w337:refnum<k21>, "error out"=w336:errorcluster)  [unwired: 12 in]
            n136 = call <vilib>:"DAQmx Stop Task.vi"("task/channels in"=w337, "error in"=w336) -> ("task out"=w338:refnum<k21>, "error out"=w339:errorcluster)  [unwired: 12 in]
            n137 = call <vilib>:"DAQmx Clear Task.vi"("task in"=w338, "error in"=w339) -> ("error out"=w340:errorcluster)  [unwired: 13 in]
            n138 = call "Sensor Read.vi"("Error In"=w340, "Pressure Freq"=w335, "Temperature Freq"=w335, "Sampling Time"=0.5) -> ("Temperature Data"=w352:waveform(dbl)[], "Photodiode Data"=w387:waveform(dbl)[])  [unwired: 4 in, 2 out]
            n139 = call "Convert to Dynamic Data"("Array of Waveforms"=w387) -> ("Dynamic Data Type"=w388:dynamicdata)  [unwired: 3 in]
            n140 = Split 1D Array(array=w352, index=w365) -> (first subarray=w371:waveform(dbl)[], second subarray=w364:waveform(dbl)[])
            n141 = Split 1D Array(array=w364, index=w362) -> (first subarray=w356:waveform(dbl)[], second subarray=w355:waveform(dbl)[])
            n142 = Multiply(x=31213.0, y=w371) -> (x*y=w397:waveform(dbl)[])
            n143 = Multiply(x=w356, y=49.97399) -> (x*y=w361:waveform(dbl)[])
            n144 = Multiply(x=w355, y=50.092507) -> (x*y=w370:waveform(dbl)[])
            n145 = Subtract(x=w397, y=125.26) -> (x-y=w367:waveform(dbl)[])
            n146 = Subtract(x=w361, y=9.683) -> (x-y=w357:waveform(dbl)[])
            n147 = Subtract(x=w370, y=10.205) -> (x-y=w358:waveform(dbl)[])
            n148 = Insert Into Array(array=w357, index=w362, new element=w358) -> (w363:waveform(dbl)[])
            n149 = Insert Into Array(array=w367, index=w365, new element=w363) -> (w366:waveform(dbl)[])
            n150 = call "Convert to Dynamic Data2"("Array of Waveforms"=w366) -> ("Dynamic Data Type"=w374:dynamicdata)  [unwired: 3 in]
            n151 = Split Signals(w374) -> (w377:dynamicdata, w376:dynamicdata, w375:dynamicdata, w373:dynamicdata, w372:dynamicdata)  [unwired: 5 in]
            n152 = Split Signals(w388) -> (w391:dynamicdata, w393:dynamicdata, w386:dynamicdata, w385:dynamicdata, w384:dynamicdata)  [unwired: 5 in]
            n153 = call "Convert from Dynamic Data"("Dynamic Data Type"=w377) -> ("Scalar"=w390:dbl)  [unwired: 3 in]
            n154 = call "Convert from Dynamic Data2"("Dynamic Data Type"=w376) -> ("Scalar"=w389:dbl)  [unwired: 3 in]
            n155 = call "Convert from Dynamic Data3"("Dynamic Data Type"=w391) -> ("Scalar"=w392:dbl)  [unwired: 3 in]
            n156 = call "Convert from Dynamic Data4"("Dynamic Data Type"=w393) -> ("Scalar"=w394:dbl)  [unwired: 3 in]
            n157 = call "Convert from Dynamic Data8"("Dynamic Data Type"=w375) -> ("Scalar"=w381:dbl)  [unwired: 3 in]
            n158 = call "Convert from Dynamic Data9"("Dynamic Data Type"=w373) -> ("Scalar"=w382:dbl)  [unwired: 3 in]
            n159 = call "Convert from Dynamic Data10"("Dynamic Data Type"=w372) -> ("Scalar"=w383:dbl)  [unwired: 3 in]
            n160 = call "Convert from Dynamic Data5"("Dynamic Data Type"=w386) -> ("Scalar"=w380:dbl)  [unwired: 3 in]
            n161 = call "Convert from Dynamic Data6"("Dynamic Data Type"=w385) -> ("Scalar"=w379:dbl)  [unwired: 3 in]
            n162 = call "Convert from Dynamic Data7"("Dynamic Data Type"=w384) -> ("Scalar"=w378:dbl)  [unwired: 3 in]
            n163 = Bundle("Scalar"=w390, "Scalar"=w389, "Scalar"=w392, "Scalar"=w394) -> (→"Predet Sensors 2":T7)  [unwired: 1 in]
            n164 = Bundle("Scalar"=w381, "Scalar"=w382, "Scalar"=w383, "Scalar"=w380, "Scalar"=w379, "Scalar"=w378) -> (→"PDE Sensors 2":T6)  [unwired: 1 in]
          }
          frame "Predet Fire" {
            w409 = PDEState."Idle"  # PDE State
            n165 = local read "Go To Idle"() -> (w406:bool)
            n166 = local read "Abort VI"() -> (w407:bool)
            n167 = Or(x=w407, y=w406) -> (x .or. y?=w405:bool)
            n168 = call "PredetControlSequence (SubVI).vi"("Stop Button"=w405, "Predet Freq (Hz)"="Predet Freq (Hz)") -> ()  [unwired: 6 in, 4 out]
            n169 = feedback #2() -> (w412:i32)  [unwired: 1 in]
            n170 = Increment(x=w412) -> (x+1=w411:i32)
            n171 = Less?(x=w411, y="Number of Predet Fires") -> (x < y?=w414:bool)
            n172 = Select(t=w411, s=w414, f=0 ("s? t:f")) -> (s? t:f=w404:i32)
            "Predet Fire Counter" <- w404
            n173 = feedback-in #2(w404) -> ()
            n174 = Divide(x=w404, y="Number of Predet Fires") -> (x/y=→"Predet Progress":dbl)
            n175 = Select(t=PDEState."Predet Fire", s=w414, f=w409) -> (s? t:f=w408:T5)
          }
        }
      }
      event "Set_Oxygen_Pressure": Value Change {
        w415 = PDEState."Control Button"  # PDE State
        n176 = event-data() -> ()  [unwired: 1 in, 6 out]
      }
      event "Predet Fire Button": Value Change {
        n177 = event-data() -> ()  [unwired: 1 in, 1 out]
      }
      event "Abort VI": Value Change {
        n178 = event-data() -> ()  [unwired: 1 in, 1 out]
      }
      event "Go To Idle": Value Change {
        n179 = event-data() -> ()  [unwired: 1 in, 1 out]
      }
      event "PDE Fire Button": Value Change {
        n180 = event-data() -> ()  [unwired: 1 in, 1 out]
      }
      event "Test Button": Value Change {
        n181 = event-data() -> ()  [unwired: 1 in, 1 out]
      }
    }
    "PDE State" <- w2
  }
